vi "UserAuthentication.vi"(8 "Error in":errorcluster) -> (0 "Error out":errorcluster, 3 "User Data":T1 {"UserType" items=["Admin", "Operator"]})   [LabVIEW 2021]
uses:
  Controls/VIStates_UserAuthentication.ctl
  Controls/UserTypes.ctl
  Controls/UserData.ctl
panel:
  in  "DeleteUser":bool
  in  "Help":bool
  in  "EditPassword":bool
  in  "AddNewUser":bool
  in  "Password":string
  in  "User Name":string(combo)
  in  "Cancel":bool
  in  "Login":bool
  # "User Authentication"
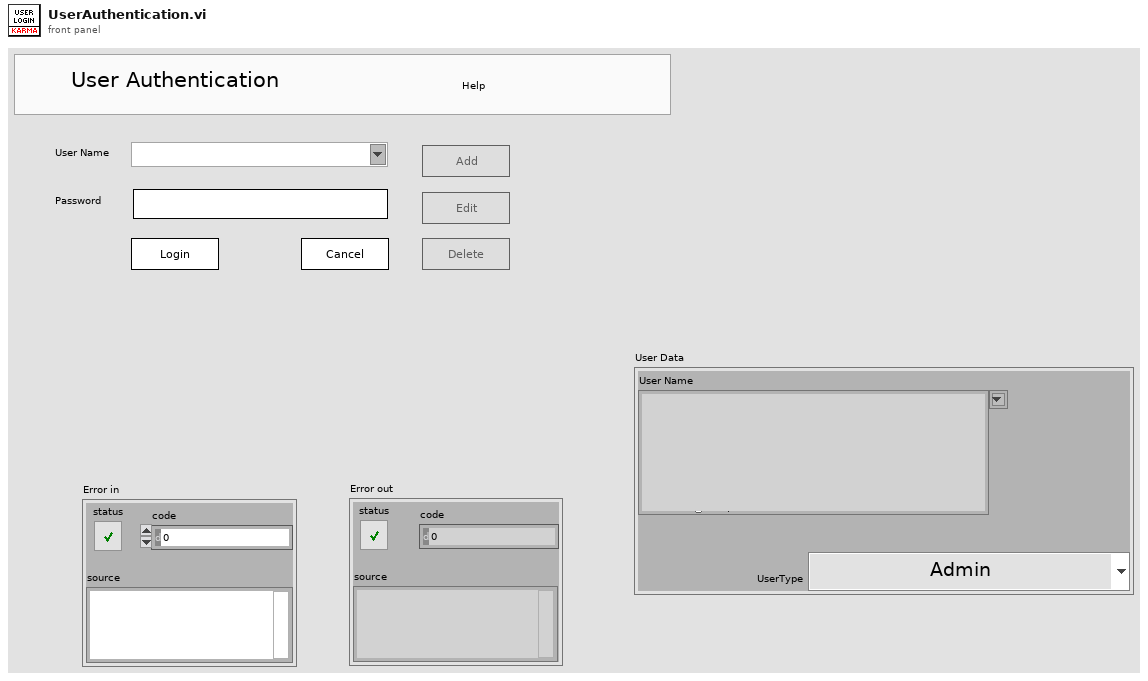
[diagram p1: front panel]
types:
  T1 = typedef "UserData.ctl" = cluster{"User Name":string, "ValidUser?(F)":bool, "UserType":T2}
  T2 = typedef "UserTypes.ctl" = u16
  T3 = typedef "VIStates_UserAuthentication.ctl" = enum16{"Poll", "Initialize", "SearchUserData", "PasswordLookup", "Validate", "UpdateUserInfo", "AddNewUser", "EditPassword", "DeleteUser", "Error", "Exit"}
  T4 = cluster{"User Info Array out":string[][], "SelectedUserName":string, "SelectedUserData":string[], "CurrentPassword":string}
  T5 = enum8{"Enabled", "Disabled", "Disabled and Grayed Out"}
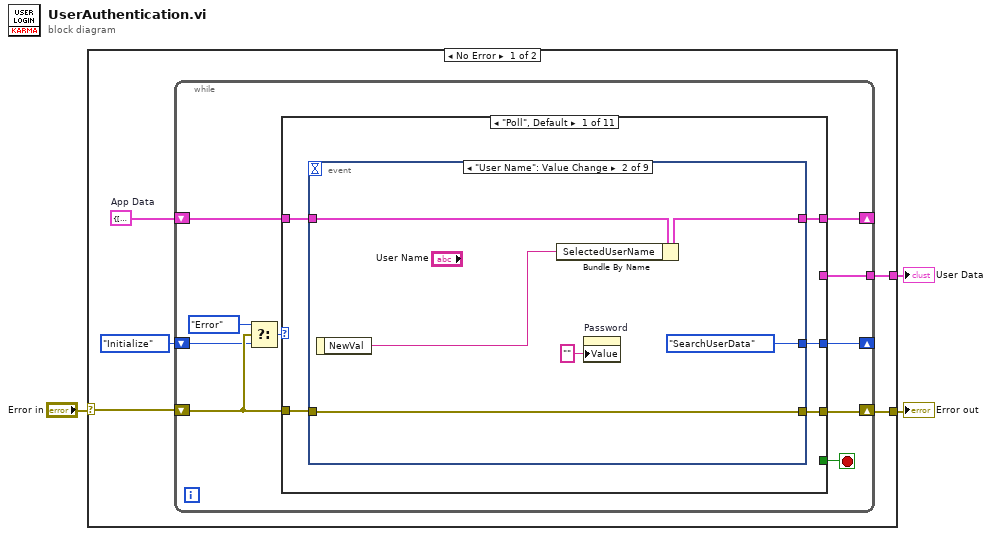
[diagram p0: block diagram]
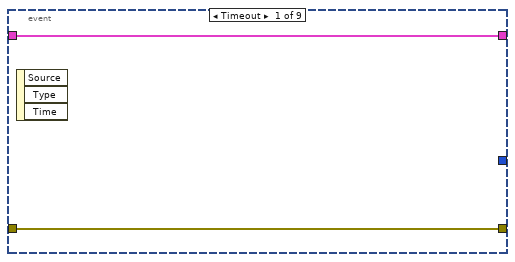
[diagram p2: hidden frame]
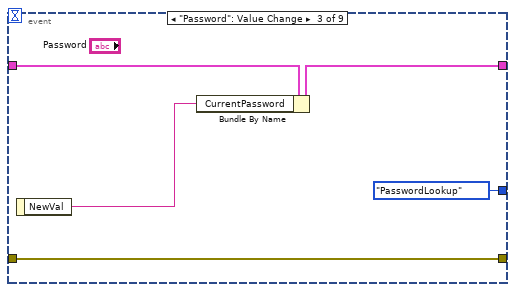
[diagram p3: hidden frame]
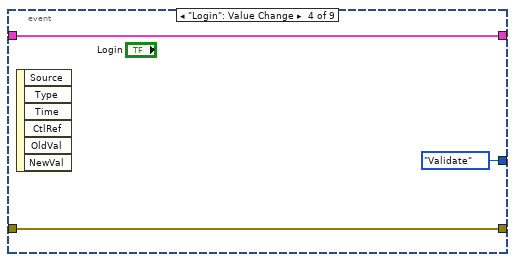
[diagram p4: hidden frame]
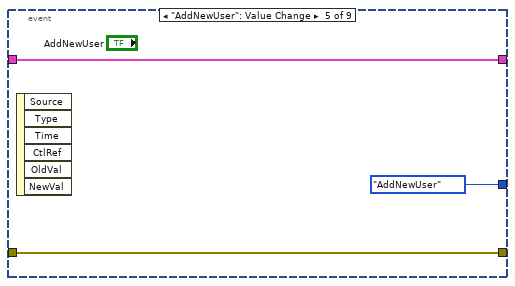
[diagram p5: hidden frame]
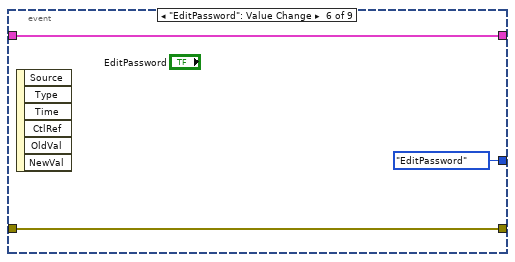
[diagram p6: hidden frame]
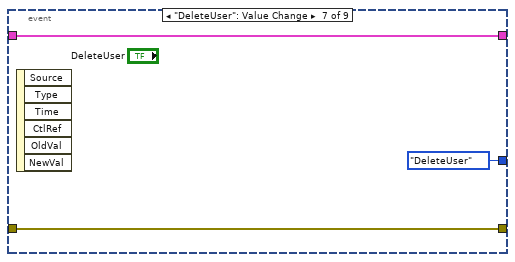
[diagram p7: hidden frame]
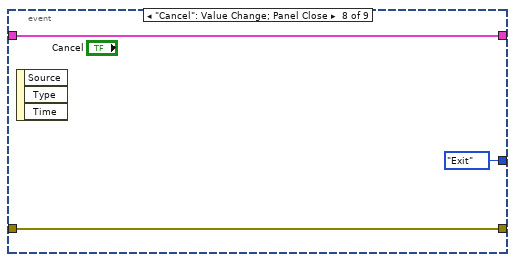
[diagram p8: hidden frame]
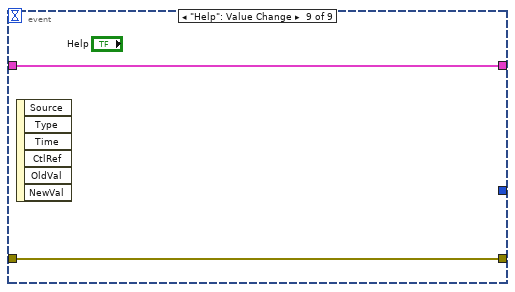
[diagram p9: hidden frame]
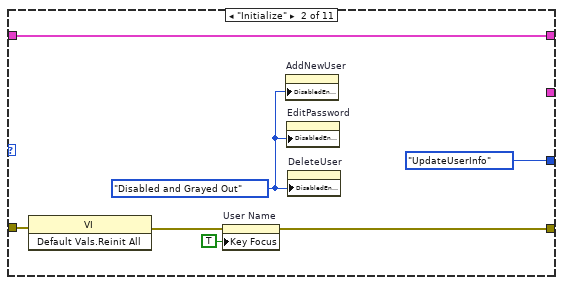
[diagram p10: hidden frame]
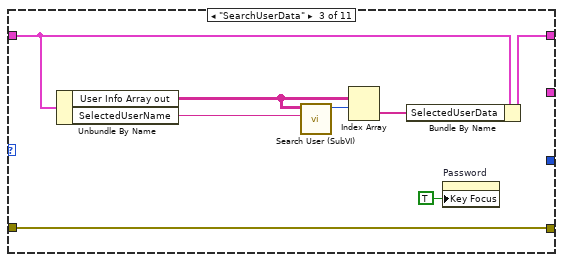
[diagram p11: hidden frame]
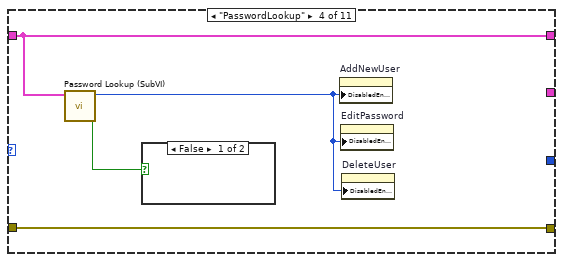
[diagram p12: hidden frame]
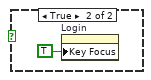
[diagram p13: hidden frame]
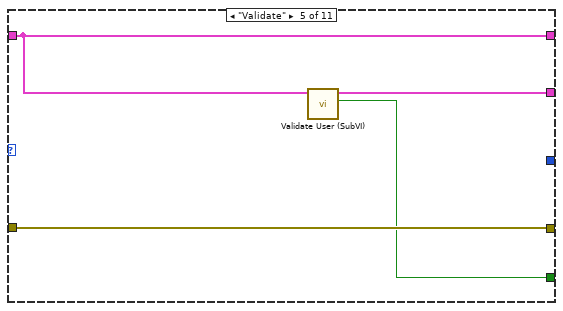
[diagram p14: hidden frame]
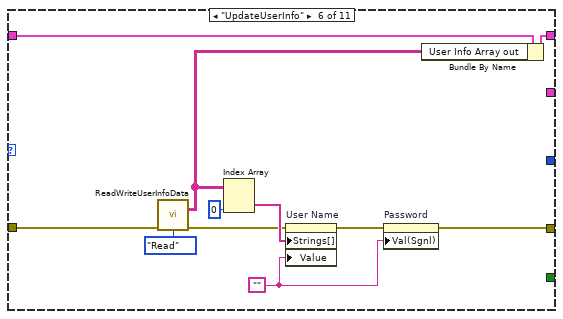
[diagram p15: hidden frame]
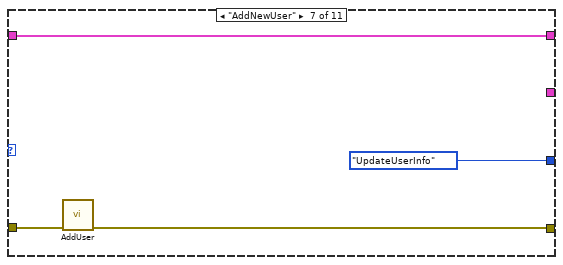
[diagram p16: hidden frame]
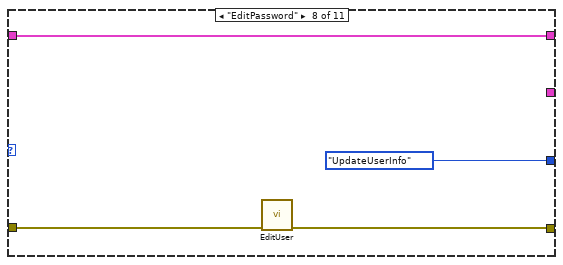
[diagram p17: hidden frame]
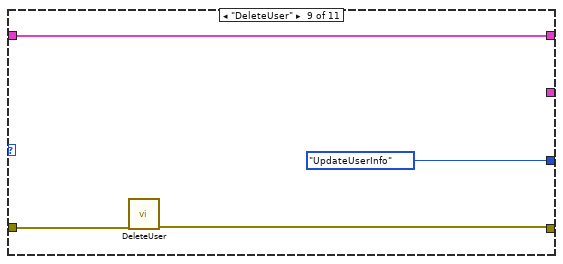
[diagram p18: hidden frame]
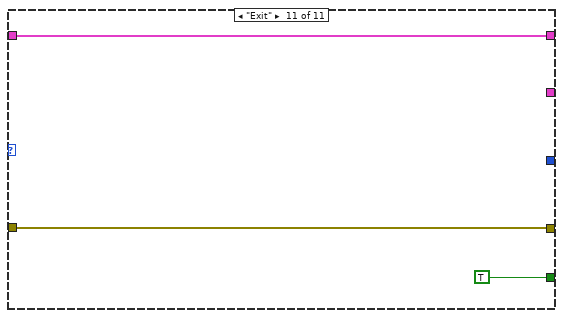
[diagram p20: hidden frame]
diagram:
  n1 = case shown="No Error" "Error in" {
    selector: "Error in" -> [w4 w106]
    tunnel: [w7 w106] -> w3
    tunnel: [w5 _] -> w2
    frame No Error {
      w6 = T4 {"User Info Array out"=[], "SelectedUserName"="", "SelectedUserData"=[], "CurrentPassword"=""}  # App Data
      n2 = while {
        shift-right: [w17] -> _
        shift-left: VIStates_UserAuthentication."Initialize" -> [w11]
        shift-right: [w16] -> _
        shift-left: w6 -> [w15]
        tunnel: [w14] -> w5
        shift-right: [w18] -> w7
        shift-left: w4 -> [w12]
        stop <- w13 stop-if-true
        n3 = Select(t=VIStates_UserAuthentication."Error", s=w12, f=w11) -> (s? t:f=w9:T3)
        n4 = case shown="\"Poll\", Default" w9 {
          tunnel: w12 -> [w23 w59 w68 w72 w77 w84 w92 w96 w100 w102 w105]
          tunnel: [w22 w54 w68 w72 w77 w83 w91 w95 w98 w102 w105] -> w18
          tunnel: [w21 VIStates_UserAuthentication."UpdateUserInfo" _ _ _ _ VIStates_UserAuthentication."UpdateUserInfo" VIStates_UserAuthentication."UpdateUserInfo" VIStates_UserAuthentication."UpdateUserInfo" _ _] -> w17
          tunnel: [w19 w58 w63 w71 w76 w79 w90 w94 w99 w101 w104] -> w16
          tunnel: w15 -> [w20 w58 w67 w71 w76 w88 w90 w94 w99 w101 w104]
          tunnel: [_ _ _ _ w75 _ _ _ _ _ _] -> w14
          tunnel: [_ _ _ _ w74 _ _ _ _ _ TRUE] -> w13
          frame "Poll", Default {
            n5 = event shown="[1] \"User Name\": Value Change" {
              selector: _ -> [_ _ _ _ _ _ _ _ _]
              dyn-events: _ -> [_ _ _ _ _ _ _ _ _]
              timeout: _ -> [_ _ _ _ _ _ _ _ _]
              tunnel: w23 -> [w25 w31 w36 w39 w42 w45 w48 w51 w53]
              tunnel: [w25 w31 w36 w39 w42 w45 w48 w51 w53] -> w22
              tunnel: [_ VIStates_UserAuthentication."SearchUserData" VIStates_UserAuthentication."PasswordLookup" VIStates_UserAuthentication."Validate" VIStates_UserAuthentication."AddNewUser" VIStates_UserAuthentication."EditPassword" VIStates_UserAuthentication."DeleteUser" VIStates_UserAuthentication."Exit" _] -> w21
              tunnel: [w24 w28 w33 w38 w40 w44 w47 w50 w52] -> w19
              tunnel: w20 -> [w24 w29 w34 w38 w40 w44 w47 w50 w52]
              event Timeout {
                n6 = event-data() -> ()  [unwired: 1 in, 3 out]
              }
              event "User Name": Value Change {
                n7 = event-data() -> ("NewVal"=w27:string)  [unwired: 1 in]
                n8 = Bundle By Name(cluster=w29, "SelectedUserName"=w27) -> (w28:T4)
                n9 = property on="Password" class="Str"("Value"="" ("Password")) -> ()  [unwired: 2 in, 2 out]
              }
              event "Password": Value Change {
                n10 = event-data() -> ("NewVal"=w32:string)  [unwired: 1 in]
                n11 = Bundle By Name(cluster=w34, "CurrentPassword"=w32) -> (w33:T4)
              }
              event "Login": Value Change {
                n12 = event-data() -> ()  [unwired: 1 in, 6 out]
              }
              event "AddNewUser": Value Change {
                n13 = event-data() -> ()  [unwired: 1 in, 6 out]
              }
              event "EditPassword": Value Change {
                n14 = event-data() -> ()  [unwired: 1 in, 6 out]
              }
              event "DeleteUser": Value Change {
                n15 = event-data() -> ()  [unwired: 1 in, 6 out]
              }
              event "Cancel": Value Change; Panel Close {
                n16 = event-data() -> ()  [unwired: 1 in, 3 out]
              }
              event "Help": Value Change {
                n17 = event-data() -> ()  [unwired: 1 in, 6 out]
              }
            }
          }
          frame "Initialize" {
            w60 = T5."Disabled and Grayed Out" ("Disabled")
            n18 = invoke class="VI" method="Default Vals.Reinit All"(error in=w59) -> (error out=w55:errorcluster)  [unwired: 2 in, 2 out]
            n19 = property on="User Name" class="CmbBox"(error in=w55, "Key Focus"=TRUE) -> (error out=w54:errorcluster)  [unwired: 1 in, 1 out]
            n20 = property on="AddNewUser" class="Bool"("DisabledEnum"=w60) -> ()  [unwired: 2 in, 2 out]
            n21 = property on="EditPassword" class="Bool"("DisabledEnum"=w60) -> ()  [unwired: 2 in, 2 out]
            n22 = property on="DeleteUser" class="Bool"("DisabledEnum"=w60) -> ()  [unwired: 2 in, 2 out]
          }
          frame "SearchUserData" {
            n23 = Unbundle By Name(w67) -> ("User Info Array out"=w65:string[][], "SelectedUserName"=w66:string)
            n24 = call "Search User (SubVI).vi"("SelectedUserName"=w66, "User Info Array in"=w65) -> ("index of element"=w64:i32)  [unwired: 9 in]
            n25 = Index Array(array=w65, index (row)=w64) -> (element=w62:string[])  [unwired: 1 in]
            n26 = Bundle By Name(cluster=w67, "SelectedUserData"=w62) -> (w63:T4)
            n27 = property on="Password" class="Str"("Key Focus"=TRUE) -> ()  [unwired: 2 in, 2 out]
          }
          frame "PasswordLookup" {
            n28 = call "Password Lookup (SubVI).vi"("App Data"=w71) -> ("Boolean"=w69:bool, "Disabled"=w70:T5)  [unwired: 9 in]
            n29 = case shown="False" w69 {
              frame False {
              }
              frame True {
                n30 = property on="Login" class="Bool"("Key Focus"=TRUE) -> ()  [unwired: 2 in, 2 out]
              }
            }
            n31 = property on="AddNewUser" class="Bool"("DisabledEnum"=w70) -> ()  [unwired: 2 in, 2 out]
            n32 = property on="EditPassword" class="Bool"("DisabledEnum"=w70) -> ()  [unwired: 2 in, 2 out]
            n33 = property on="DeleteUser" class="Bool"("DisabledEnum"=w70) -> ()  [unwired: 2 in, 2 out]
          }
          frame "Validate" {
            n34 = call "Validate User (SubVI).vi"("App Data"=w76) -> ("Exit?"=w74:bool, "User Data"=w75:T1)  [unwired: 9 in]
          }
          frame "UpdateUserInfo" {
            w82 = "" ("Value (Signaling)")
            n35 = call "ReadWriteUserInfoData.vi"("Error in (no error)"=w84, "Operation"=enum16{"Write", "Read"}."Read") -> ("User Info Array out"=w78:string[][], "Error out"=w81:errorcluster)  [unwired: 11 in, 1 out]
            n36 = Index Array(array=w78, index (col)=0 ("disabled index (col)")) -> (element=w87:string[])  [unwired: 1 in]
            n37 = property on="User Name" class="CmbBox"(error in=w81, "Strings[]"=w87, "Value"=w82) -> (error out=w80:errorcluster)  [unwired: 1 in, 1 out]
            n38 = property on="Password" class="Str"(error in=w80, "Val(Sgnl)"=w82) -> (error out=w83:errorcluster)  [unwired: 1 in, 1 out]
            n39 = Bundle By Name(cluster=w88, "User Info Array out"=w78) -> (w79:T4)
          }
          frame "AddNewUser" {
            n40 = call "AddUser.vi"("error in (no error)"=w92) -> ("error out"=w91:errorcluster)  [unwired: 10 in]
          }
          frame "EditPassword" {
            n41 = call "EditUser.vi"("error in (no error)"=w96) -> ("error out"=w95:errorcluster)  [unwired: 14 in]
          }
          frame "DeleteUser" {
            n42 = call "DeleteUser.vi"("error in (no error)"=w100) -> ("error out"=w98:errorcluster)  [unwired: 10 in]
          }
          frame "Error" {
          }
          frame "Exit" {
          }
        }
      }
    }
    frame Error {
    }
  }
  "User Data" <- w2
  "Error out" <- w3
